vi "Find Tests.vi"(8 "error in (no error)":errorcluster, 10 "Project Refnum":refnum<vi>, 11 "Test Discoverer in":refnum<class "Test Discoverer.lvclass">) -> (0 "error out":errorcluster, 2 "Test Cases":refnum<class "Test Case.lvclass">[](array[class]), 3 "Test Discoverer out":refnum<class "Test Discoverer.lvclass">)   [LabVIEW 2017, in "Test Discoverer.lvclass"]
doc: "Finds the tests available from the specified project refnum."
uses:
  Test Discoverer.lvclass
  Test Case/Test Case.lvclass
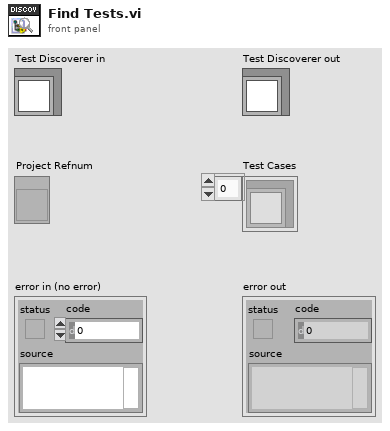
[diagram p1: front panel]
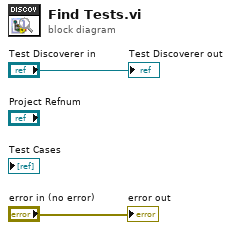
[diagram p0: block diagram]
diagram:
  "error out" <- "error in (no error)"
  "Test Discoverer out" <- "Test Discoverer in"
